vi "fgv_PXIe-2530_config.vi"(7 "cmd":T3, 11 "config":T1={"visa"="PXI1Slot2", "topology"="Configured Topology", "relay name"="k0", "relay action"=21} {"relay action" items=["Open Relay"=20, "Close Relay"=21]}) -> (3 "config 2":T1={"visa"="PXI1Slot2", "topology"="Configured Topology", "relay name"="k0", "relay action"=21} {"relay action" items=["Open Relay"=20, "Close Relay"=21]})   [LabVIEW 2021]
uses:
  ctrl/rw.ctl
  ctrl/PXIe-2530_cfg.ctl
  <instrlib>/niSwitch/niSwitch.llb/niSwitch Topologies.ctl
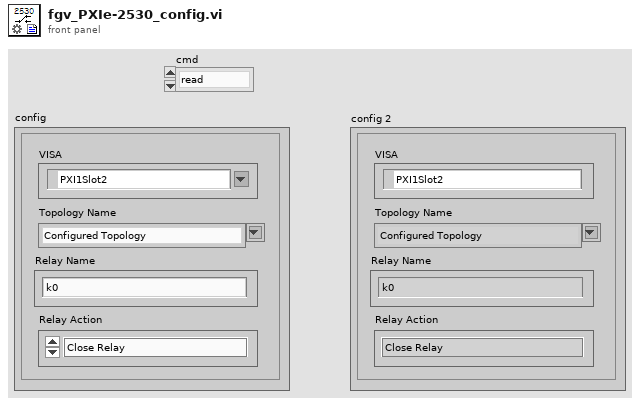
[diagram p1: front panel]
types:
  T1 = typedef "PXIe-2530_cfg.ctl" = cluster{"visa":refnum<k15>, "topology":T2, "relay name":string, "relay action":i32}
  T2 = typedef "niSwitch Topologies.ctl" = string
  T3 = typedef "rw.ctl" = enum16{"read", "write"}
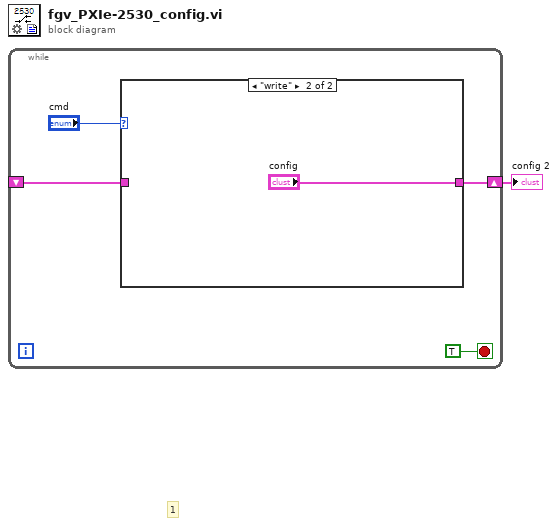
[diagram p0: block diagram]
diagram:
  # "1"
  n1 = while {
    shift-right: [w3] -> w1
    shift-left: _ -> [w2]
    stop <- TRUE stop-if-true
    n2 = case shown="\"write\"" "cmd" {
      tunnel: [w6 "config"] -> w3
      tunnel: w2 -> [w6 _]
      frame "read", Default {
      }
      frame "write" {
      }
    }
  }
  "config 2" <- w1
